vi "計時器+自保持.vi"(4 "時間設定":dbl format="%#.6f", 6 "動作":bool) -> (0 "時間到":bool, 2 "計數時間":dbl format="%.2f", 3 "開始時間":dbl format="%.2f")   [LabVIEW 2015]
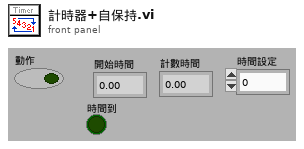
[diagram p1: front panel]
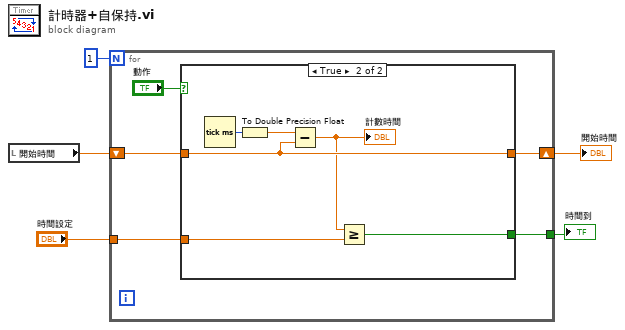
[diagram p0: block diagram]
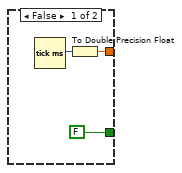
[diagram p2: hidden frame]
diagram:
  n1 = local read "開始時間"() -> (w3:dbl)
  n2 = for {
    N: 1 -> [_]
    shift-right: [w9] -> w4
    shift-left: w3 -> [w10]
    tunnel: "時間設定" -> [w7]
    tunnel: [w6] -> w1
    n3 = case shown="True" "動作" {
      tunnel: w10 -> [_ w19]
      tunnel: [w13 w19] -> w9
      tunnel: w7 -> [_ w15]
      tunnel: [FALSE w14] -> w6
      frame False {
        n4 = Tick Count (ms)() -> (millisecond timer value=w11:u32)
        n5 = To Double Precision Float(number=w11) -> (double precision float=w13:dbl)
      }
      frame True {
        n6 = Tick Count (ms)() -> (millisecond timer value=w18:u32)
        n7 = To Double Precision Float(number=w18) -> (double precision float=w17:dbl)
        n8 = Subtract(x=w17, y=w19) -> (x-y=w16:dbl)
        "計數時間" <- w16
        n9 = Greater Or Equal?(x=w16, y=w15) -> (x >= y?=w14:bool)
      }
    }
  }
  "開始時間" <- w4
  "時間到" <- w1
